vi "Handle Process Error.vi"(8 "error in (no error)":errorcluster, 10 "Location":string, 11 "Process In":refnum<class "Process.lvclass">) -> (0 "error out":errorcluster, 3 "Process Out":refnum<class "Process.lvclass">)   [LabVIEW 2020, in "Process.lvclass"]
doc: "Send any error to the Error Handler Interface configured using the Set Error Handler.vi method. This method is used by the framework in the process loop, but may also be used to send errors that cannot be handled locally to the centralized error handler."
uses:
  Process.lvclass
  Process.lvclass/Process.ctl
  Error Handler Interface/Error Handler Interface.lvclass
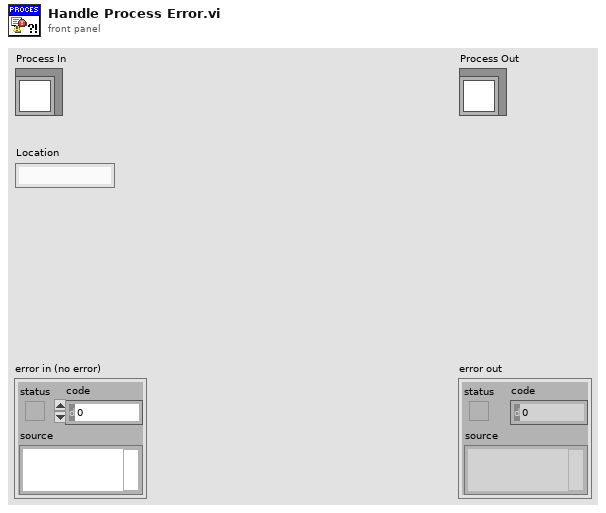
[diagram p1: front panel]
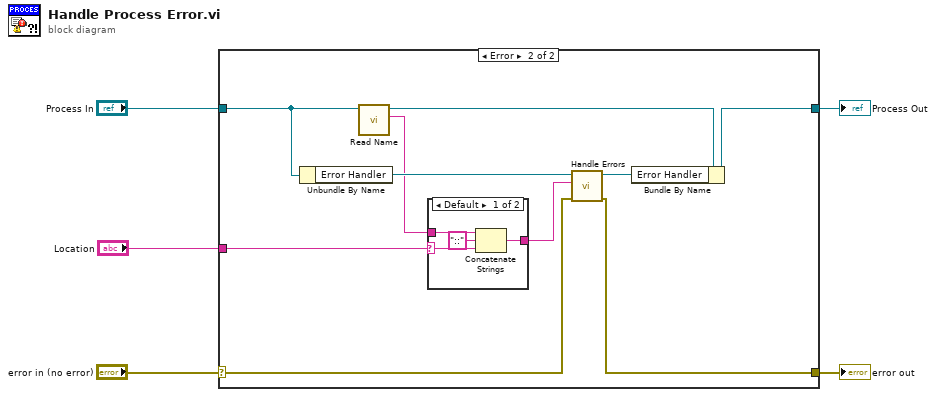
[diagram p0: block diagram]
diagram:
  n1 = case shown="Error" "error in (no error)" {
    selector: "error in (no error)" -> [w6 w15]
    tunnel: [w6 w14] -> w4
    tunnel: [w7 w16] -> w2
    tunnel: "Process In" -> [w7 w13]
    tunnel: "Location" -> [_ w8]
    frame No Error {
    }
    frame Error {
      n2 = Unbundle By Name(w13) -> ("Error Handler"=w17:refnum<class "Error Handler Interface.lvclass">)
      n3 = call-dynamic "Read Name.vi"("Process In"=w13) -> ("Qualified Name"=w11:string, "Process Out"=w12:refnum<class "Process.lvclass">)  [unwired: 7 in, 2 out]
      n4 = case shown="Default" w8 {
        selector: w8 -> [w19 _]
        tunnel: w11 -> [w21 w22]
        tunnel: [w20 w22] -> w9
        frame Default {
          n5 = Concatenate Strings(w21, "::" ("string"), w19) -> (w20:string)
        }
        frame "" {
        }
      }
      n6 = call-dynamic "Handle Errors.vi"("error in (no error)"=w15, "Location"=w9, "Error Handler Interface In"=w17) -> ("error out"=w14:errorcluster, "Error Handler Interface Out"=w10:refnum<class "Error Handler Interface.lvclass">)  [unwired: 7 in]
      n7 = Bundle By Name(cluster=w12, "Error Handler"=w10) -> (w16:refnum<class "Process.lvclass">)
    }
  }
  "error out" <- w4
  "Process Out" <- w2
